vi "InitialTrayStatus.vi"(8 "error in (no error)":errorcluster, 11 "AI in":refnum<class "AI.lvclass">) -> (0 "error out":errorcluster, 3 "AI out":refnum<class "AI.lvclass">)   [LabVIEW 2019, in "AI.lvclass"]
uses:
  AI.lvclass
  Function/TraySet Folder/global/Tray_ArrAndData.vi
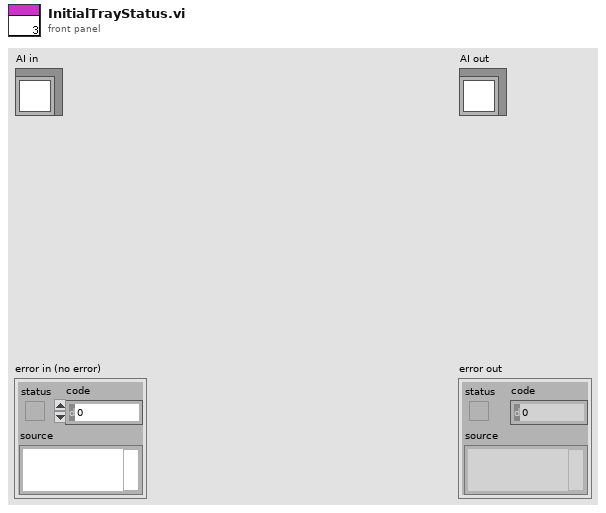
[diagram p1: front panel]
types:
  T1 = cluster{"XY_BTray":cluster{"X":i32, "Y":i32}, "Initial color":u32, "FinalColor":u32}
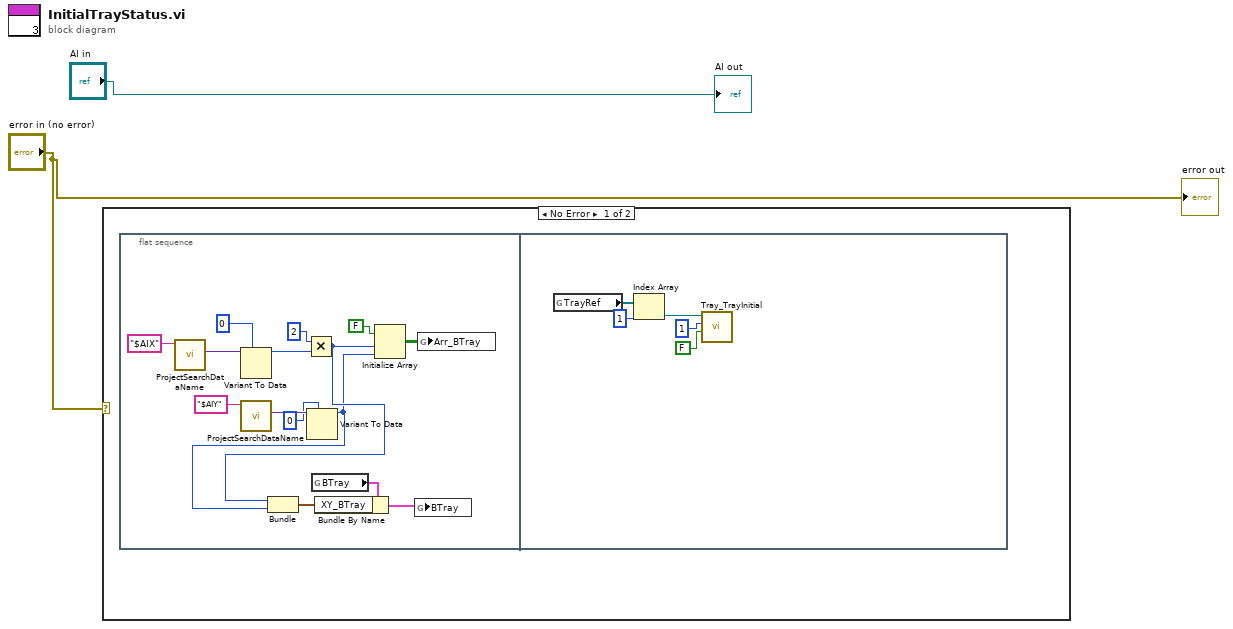
[diagram p0: block diagram]
diagram:
  n1 = case shown="No Error" "error in (no error)" {
    frame No Error {
      n2 = flat-sequence {
        frame #0 {
          n3 = call "ProjectSearchDataName.vi"("element"="$AIX") -> ("variant"=w14:variant)  [unwired: 7 in, 3 out]
          n4 = Variant To Data(type=0, Variant=w14) -> (data=w11:i32)  [unwired: 1 in, 1 out]
          n5 = call "ProjectSearchDataName.vi"("element"="$AIY") -> ("variant"=w15:variant)  [unwired: 7 in, 3 out]
          n6 = Multiply(x=2, y=w11) -> (x*y=w4:i32)
          n7 = Variant To Data(type=0, Variant=w15) -> (data=w3:i32)  [unwired: 1 in, 1 out]
          n8 = Bundle(w4, w3) -> (w5:cluster{i32, i32})  [unwired: 1 in]
          n9 = global read "Tray_ArrAndData.vi" "BTray"() -> (w7:T1)
          n10 = Bundle By Name(cluster=w7, "XY_BTray"=w5) -> (w6:T1)
          n11 = Initialize Array(FALSE, w4, w3) -> (w9:bool[][])
          n12 = global write "Tray_ArrAndData.vi" "BTray"(w6) -> ()
          n13 = global write "Tray_ArrAndData.vi" "Arr_BTray"(w9) -> ()
        }
        frame #1 {
          n14 = global read "Tray_ArrAndData.vi" "TrayRef"() -> (w21:refnum<vi>[])
          n15 = Index Array(array=w21, index=1) -> (element=w20:refnum<vi>)
          n16 = call "Tray_TrayInitial.vi"("SetColor"=FALSE, "TrayCase"=1, "TrayIn"=w20) -> ()  [unwired: 8 in, 1 out]
        }
      }
    }
    frame Error {
    }
  }
  "error out" <- "error in (no error)"
  "AI out" <- "AI in"
